vi "Acquisition Message Loop.vi"(8 "error in (no error)":errorcluster, 9 "Data Queue":refnum<queue>, 10 "Data Notifier":refnum<notifier>, 11 "Message Queues":T1) -> (0 "error out":errorcluster)   [LabVIEW 2017, in "Acquisition.lvlib"]
doc: "Message loop for handling messages pertaining to the acquisition of data from the hardware."
uses:
  Acquisition.lvlib
  support/Message Queue/All Message Queues.ctl
  support/Message Queue/Message Cluster.ctl
  Hardware Configuration.ctl
  Signal Type.ctl
  Settings/Terminal Configuration.ctl
  Settings/Range.ctl
  Settings/Coupling.ctl
  Settings/Sampling Clock Source.ctl
  Settings/Time Units.ctl
  Settings/Resolution.ctl
  Settings/Trigger Direction.ctl
  Settings/Trigger Source.ctl
  Settings/Quantity.ctl
  Acquisition State.ctl
  support/Active channels.vi
  support/Message Queue/Enqueue Message (Array).vi
  support/Message Queue/Enqueue Message (Single).vi
  <vilib>/Utility/error.llb/Error Cluster From Error Code.vi
  <vilib>/ErrorRing/Error Ring.xnode
  support/Message Queue/Message Queue.lvlib
  Settings/Settings.lvlib
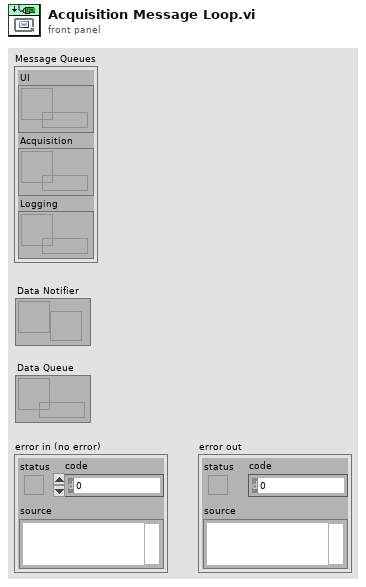
[diagram p1: front panel]
types:
  T1 = typedef "Message Queue.lvlib/All Message Queues.ctl" = cluster{"UI":refnum<queue>, "Acquisition":refnum<queue>, "Logging":refnum<queue>}
  T2 = typedef "Acquisition.lvlib/Hardware Configuration.ctl" = cluster{"VISA resource name":refnum<visa-resource-name>, "DAQ Type":T3, "Channel 1":cluster{"Acquiring":bool, "Enabled":bool, "Terminal configuration":T4, "Range":T5, "Coupling":T6}, "Channel 2":cluster{"Acquiring":bool, "Enabled":bool, "Terminal configuration":T4, "Range":T5, "Coupling":T6}, "Timing":cluster{"Sample Time [Time Units]":u32, "Actual Sample Time [s]":dbl, "Samples per Iteration":u32, "Sample Clock Source":T7, "Time Units":T8, "t0":timestamp}, "PS Parameters":cluster{"PS handle":i16, "PS Max_adc":i16, "PS Enabled Array":i16[], "PS Device Info":cluster{"Driver Version":string, "USB Version":string, "Hardware":string, "Variant":string, "Batch and Serial":string, "Cal Date":string, "Kernel Version":string, "Digital HW Version":string, "Analogue HW Version":string, "Firmware 1":string, "Firmware 2":string, "MSO":bool, "Number of Channels":i16}, "Channel 1 Buffer":refnum<data-value>, "Channel 2 Buffer":refnum<data-value>, "Resolution":T9, "USB Power":bool}, "Trigger":cluster{"Direction":T10, "Threshold [V]":dbl, "Enabled":bool, "Trigger Source":T11}, "Keithley Parameters":cluster{"Previous End / Current Start":i32, "Quantity":T12}}
  T3 = typedef "Acquisition.lvlib/Signal Type.ctl" = u16
  T4 = typedef "Settings.lvlib/Terminal Configuration.ctl" = u16
  T5 = typedef "Settings.lvlib/Range.ctl" = u16
  T6 = typedef "Settings.lvlib/Coupling.ctl" = i16
  T7 = typedef "Settings.lvlib/Sampling Clock Source.ctl" = u16
  T8 = typedef "Settings.lvlib/Time Units.ctl" = u32
  T9 = typedef "Settings.lvlib/Resolution.ctl" = i32
  T10 = typedef "Settings.lvlib/Trigger Direction.ctl" = u16
  T11 = typedef "Settings.lvlib/Trigger Source.ctl" = u16
  T12 = typedef "Settings.lvlib/Quantity.ctl" = u16
  T13 = typedef "Acquisition.lvlib/Acquisition State.ctl" = enum16{"Idle", "Acquiring"}
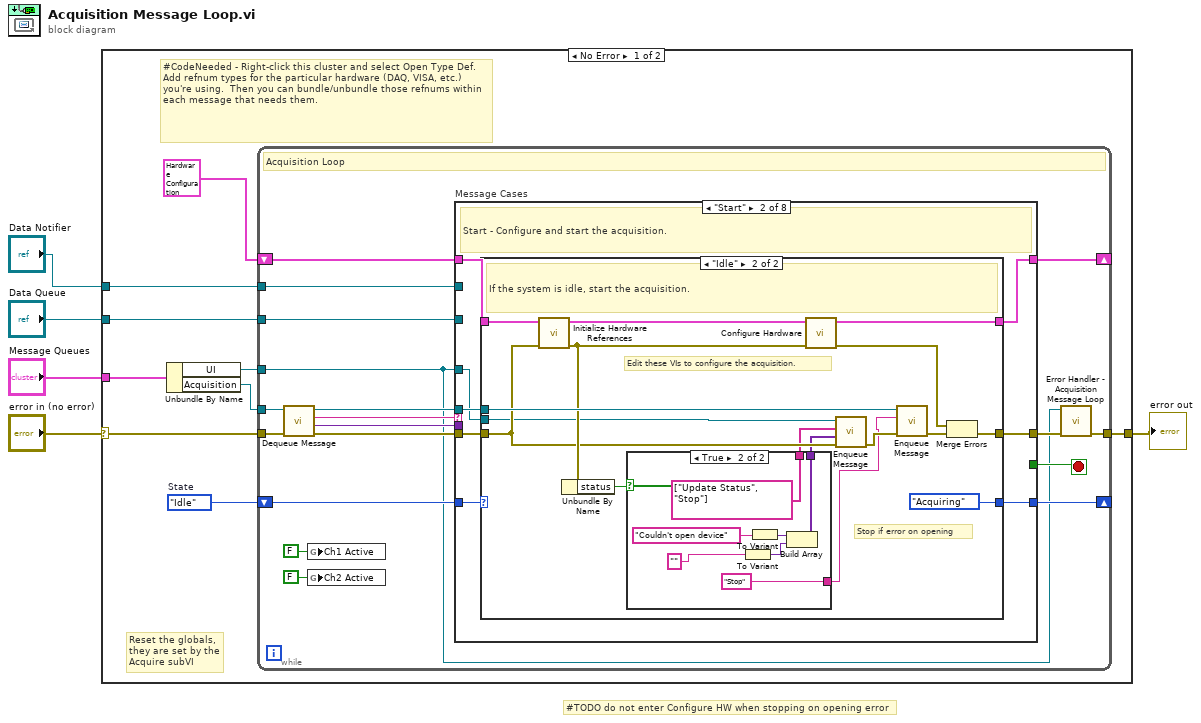
[diagram p0: block diagram]
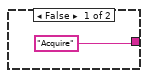
[diagram p4: hidden frame]
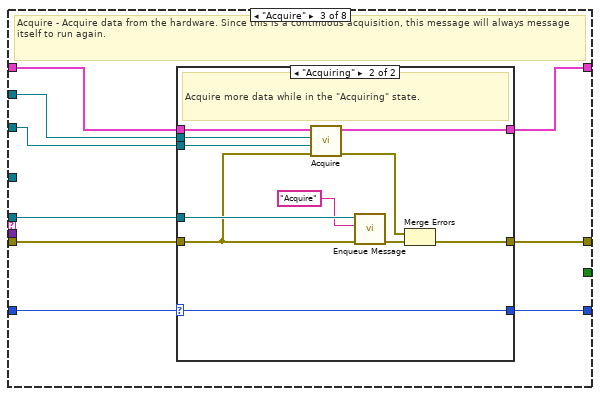
[diagram p5: hidden frame]
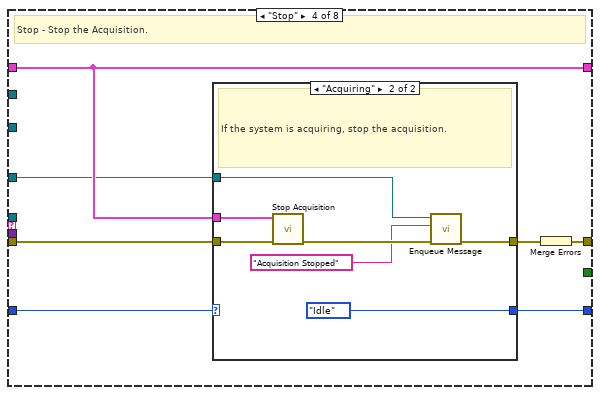
[diagram p7: hidden frame]
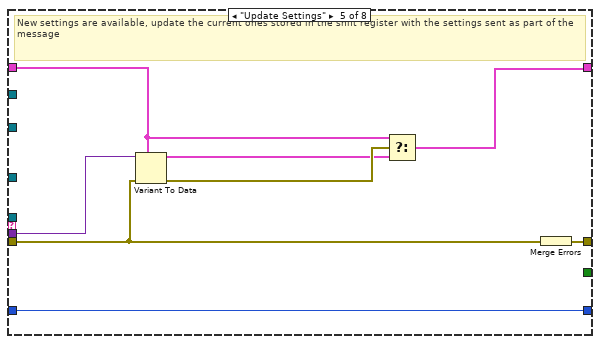
[diagram p9: hidden frame]
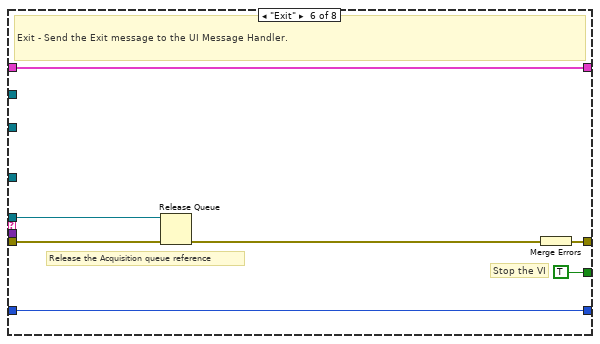
[diagram p10: hidden frame]
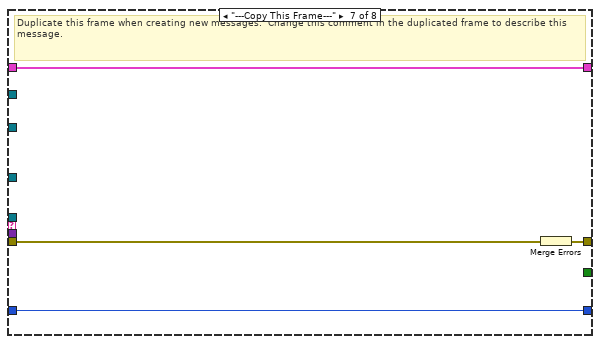
[diagram p11: hidden frame]
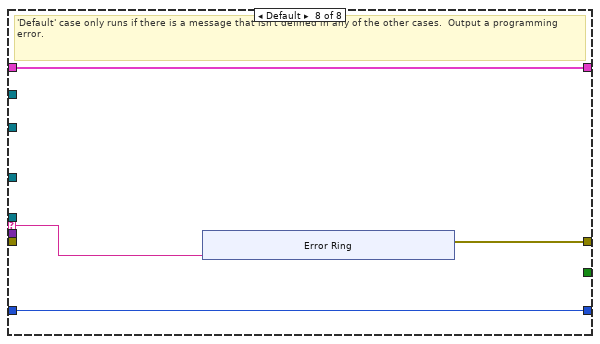
[diagram p12: hidden frame]
diagram:
  # "#TODO do not enter Configure HW when stopping on opening error"
  n1 = case shown="No Error" "error in (no error)" {
    selector: "error in (no error)" -> [w10 w140]
    tunnel: "Message Queues" -> [w14 _]
    tunnel: [w12 w140] -> w4
    tunnel: "Data Notifier" -> [w8 _]
    tunnel: "Data Queue" -> [w7 _]
    frame No Error {
      w6 = Acquisition_State."Idle"  # State
      # "Reset the globals,\nthey are set by the\nAcquire subVI"
      # "#CodeNeeded - Right-click this cluster and select Open Type Def.  Add refnum types for the particular hardware (DAQ, VISA, etc.) you're using.  Then you can bundle/unbundle those refnums within each message that needs them."
      n2 = Unbundle By Name(w14) -> ("UI"=w9:refnum<queue>, "Acquisition"=w13:refnum<queue>)
      n3 = while {
        tunnel: w13 -> [w27]
        shift-right: [w17] -> _
        shift-left: T2 {"VISA resource name"="", "DAQ Type"=0, "Channel 1"={"Acquiring"=FALSE, "Enabled"=FALSE, "Terminal configuration"=32767, "Range"=0, "Coupling"=0}, "Channel 2"={"Acquiring"=FALSE, "Enabled"=FALSE, "Terminal configuration"=0, "Range"=0, "Coupling"=0}, "Timing"={"Sample Time [Time Units]"=0, "Actual Sample Time [s]"=0.0, "Samples per Iteration"=0, "Sample Clock Source"=0, "Time Units"=0, "t0"=timestamp(0 s since 1904-01-01)}, "PS Parameters"={"PS handle"=0, "PS Max_adc"=32767, "PS Enabled Array"=[], "PS Device Info"={"Driver Version"="", "USB Version"="", "Hardware"="", "Variant"="", "Batch and Serial"="", "Cal Date"="", "Kernel Version"="", "Digital HW Version"="", "Analogue HW Version"="", "Firmware 1"="", "Firmware 2"="", "MSO"=FALSE, "Number of Channels"=0}, "Channel 1 Buffer"=refnum, "Channel 2 Buffer"=refnum, "Resolution"=0, "USB Power"=FALSE}, "Trigger"={"Direction"=0, "Threshold [V]"=0.0, "Enabled"=FALSE, "Trigger Source"=0}, "Keithley Parameters"={"Previous End / Current Start"=0, "Quantity"=0}} ("Data Cluster") -> [w18]
        tunnel: w9 -> [w19]
        tunnel: w8 -> [w26]
        tunnel: w7 -> [w25]
        shift-right: [w23] -> _
        shift-left: w6 -> [w24]
        tunnel: w10 -> [w31]
        tunnel: [w22] -> w12
        stop <- w32 stop-if-true
        # "Acquisition Loop"
        n4 = call "Dequeue Message.vi"("error in (no error)"=w31, "Message Queue"=w27) -> ("error out"=w30:errorcluster, "Message Data"=w28:variant, "Message"=w29:string, "dup Message Queue"=w20:refnum<queue>)  [unwired: 6 in]
        n5 = global write "Active channels.vi" "Ch1 Active"(FALSE ("Ch1 Active")) -> ()
        n6 = global write "Active channels.vi" "Ch2 Active"(FALSE ("Ch2 Active")) -> ()
        n7 = case "Message Cases" shown="\"Start\"" w29 {
          selector: w29 -> [_ _ _ _ _ _ _ w129]
          tunnel: w20 -> [_ w40 w78 _ _ w119 _ _]
          tunnel: w30 -> [w35 w41 w77 w99 w111 w121 w128 _]
          tunnel: [w35 w43 w79 w100 w117 w123 w126 w130] -> w21
          tunnel: w18 -> [w34 w42 w75 w97 w113 w122 w127 w132]
          tunnel: [w34 w39 w76 w97 w112 w122 w127 w132] -> w17
          tunnel: [_ _ _ _ _ TRUE _ _] -> w32
          tunnel: w28 -> [_ _ _ _ w116 _ _ _]
          tunnel: w19 -> [_ w36 _ w94 _ _ _ _]
          tunnel: w26 -> [_ _ w74 _ _ _ _ _]
          tunnel: w25 -> [_ _ w73 _ _ _ _ _]
          tunnel: w24 -> [w33 w37 w71 w96 w110 w118 w125 w131]
          tunnel: [w33 w38 w72 w95 w110 w118 w125 w131] -> w23
          frame "Initialize" {
            # "Initialize  - Initialize is currently a no-op.  The hardware initialization takes place in the 'Start' message."
          }
          frame "Start" {
            # "Start - Configure and start the acquisition."
            n8 = case shown="\"Idle\"" w37 {
              selector: w37 -> [w44 _]
              tunnel: [w45 w62] -> w43
              tunnel: w42 -> [w46 w61]
              tunnel: w41 -> [w45 w53]
              tunnel: w40 -> [_ w59]
              tunnel: [w46 w56] -> w39
              tunnel: [w44 Acquisition_State."Acquiring" ("Acquisition State")] -> w38
              tunnel: w36 -> [_ w51]
              frame "Acquiring" {
                # "The system is already acquiring. Ignore the \"Start\" message."
              }
              frame "Idle" {
                # "Stop if error on opening"
                # "Edit these VIs to configure the acquisition."
                # "If the system is idle, start the acquisition."
                n9 = call "Initialize Hardware References.vi"("error in (no error)"=w53, "Hardware Resources in"=w61) -> ("error out"=w54:errorcluster, "Hardware Resources out"=w57:T2)  [unwired: 8 in]
                n10 = Unbundle By Name(w54) -> ("status"=w50:bool)
                n11 = case shown="True" w50 {
                  tunnel: [_ string[] ["Update Status", "Stop"] ("Message Array")] -> w49
                  tunnel: [_ w67] -> w48
                  tunnel: ["Acquire" ("Message") "Stop" ("Message")] -> w47
                  frame False {
                  }
                  frame True {
                    n12 = To Variant(anything="" ("Message")) -> (Variant=w65:variant)
                    n13 = To Variant(anything="Couldn't open device" ("Message")) -> (Variant=w66:variant)
                    n14 = Build Array(w66, w65) -> (w67:variant[])
                  }
                }
                n15 = call "Configure Hardware.vi"("error in (no error)"=w54, "Hardware Resources in"=w57) -> ("error out"=w58:errorcluster, "Hardware Resources out"=w56:T2)  [unwired: 8 in]
                n16 = call-poly "Enqueue Message.vi"("error in (no error)"=w53, "Message Data Array"=w48, "Message Array"=w49, "Message Queue"=w51) -> ("error out"=w52:errorcluster)  [unwired: 6 in, 1 out]
                n17 = call-poly "Enqueue Message.vi"("error in (no error)"=w52, "Message"=w47, "Message Queue"=w59) -> ("error out"=w60:errorcluster)  [unwired: 7 in, 1 out]
                n18 = Merge Errors(w58, w60) -> (w62:errorcluster)
              }
            }
          }
          frame "Acquire" {
            # "Acquire - Acquire data from the hardware. Since this is a continuous acquisition, this message will always message itself to run again."
            n19 = case shown="\"Acquiring\"" w71 {
              selector: w71 -> [w80 w84]
              tunnel: [w81 w93] -> w79
              tunnel: w78 -> [_ w91]
              tunnel: w77 -> [w81 w83]
              tunnel: [w82 w89] -> w76
              tunnel: w75 -> [w82 w88]
              tunnel: w74 -> [_ w86]
              tunnel: w73 -> [_ w85]
              tunnel: [w80 w84] -> w72
              frame "Idle" {
                # "Ignore \"Acquire\" messages when the acquisition is idle."
              }
              frame "Acquiring" {
                # "Acquire more data while in the \"Acquiring\" state."
                n20 = call "Acquire.vi"("error in (no error)"=w83, "Data Queue"=w85, "Data Notifier"=w86, "Hardware Resources in"=w88) -> ("error out"=w90:errorcluster, "Hardware Resources out"=w89:T2)  [unwired: 6 in]
                n21 = call-poly "Enqueue Message.vi"("error in (no error)"=w83, "Message"="Acquire", "Message Queue"=w91) -> ("error out"=w92:errorcluster)  [unwired: 7 in, 1 out]
                n22 = Merge Errors(w90, w92) -> (w93:errorcluster)
              }
            }
          }
          frame "Stop" {
            # "Stop - Stop the Acquisition."
            n23 = case shown="\"Acquiring\"" w96 {
              selector: w96 -> [w101 _]
              tunnel: w99 -> [w102 w109]
              tunnel: [w102 w105] -> w98
              tunnel: w97 -> [_ w107]
              tunnel: [w101 Acquisition_State."Idle" ("State")] -> w95
              tunnel: w94 -> [_ w104]
              frame "Idle" {
                # "The system is already idle. Ignore the \"Stop\" message."
              }
              frame "Acquiring" {
                # "If the system is acquiring, stop the acquisition."
                n24 = call "Stop Acquisition.vi"("error in (no error)"=w109, "Hardware Resources in"=w107) -> ("error out"=w108:errorcluster)  [unwired: 9 in]
                n25 = call-poly "Enqueue Message.vi"("error in (no error)"=w108, "Message"="Acquisition Stopped", "Message Queue"=w104) -> ("error out"=w105:errorcluster)  [unwired: 7 in, 1 out]
              }
            }
            n26 = Merge Errors(w98) -> (w100:errorcluster)
          }
          frame "Update Settings" {
            # "New settings are available, update the current ones stored in the shift register with the settings sent as part of the message"
            n27 = Variant To Data(error in=w111, type=w113, Variant=w116) -> (data=w114:T2, error out=w115:errorcluster)
            n28 = Select(t=w113, s=w115, f=w114) -> (s? t:f=w112:T2)
            n29 = Merge Errors(w111) -> (w117:errorcluster)
          }
          frame "Exit" {
            # "Release the Acquisition queue reference"
            # "Stop the VI"
            # "Exit - Send the Exit message to the UI Message Handler."
            n30 = Release Queue(queue=w119, error in (no error)=w121) -> (error out=w120:errorcluster)  [unwired: 1 in, 2 out]
            n31 = Merge Errors(w120) -> (w123:errorcluster)
          }
          frame "---Copy This Frame---" {
            # "Duplicate this frame when creating new messages.  Change this comment in the duplicated frame to describe this message."
            n32 = Merge Errors(w128) -> (w126:errorcluster)
          }
          frame Default {
            # "'Default' case only runs if there is a message that isn't defined in any of the other cases.  Output a programming error."
            n33 = xnode "Error Ring"("parameter 0"=w129) -> ("error out"=w130:errorcluster)
          }
        }
        n34 = call "Error Handler - Acquisition Message Loop.vi"("error in (no error)"=w21, "Message Queue"=w19) -> ("dup error in"=w22:errorcluster)  [unwired: 8 in, 1 out]
      }
    }
    frame Error {
    }
  }
  "error out" <- w4
